vi "7FFT矩形窗校正子程序.vi"(6 "averaging parameters":T1={"averaging mode"=enum."No averaging", "weighting mode"=enum."Exponential", "number of averages"=10}, 7 "time signal":waveform(dbl) caption="时间信号") -> (0 "FFT幅值":cluster{"f0":dbl, "df":dbl, "magnitude":dbl[]}(graph), 2 "FFT相位":cluster{"f0":dbl, "df":dbl, "phase":dbl[]}(graph), 3 "频率":dbl)   [LabVIEW 2017]
uses:
  <vilib>/Analysis/4window.llb/windowTd.ctl
  <vilib>/measure/maspectr.llb/FFT Spectrum (Mag-Phase) for 1 Chan.vi
  <vilib>/measure/NI_MAPro.lvlib
  <vilib>/Analysis/NI_AALPro.lvlib
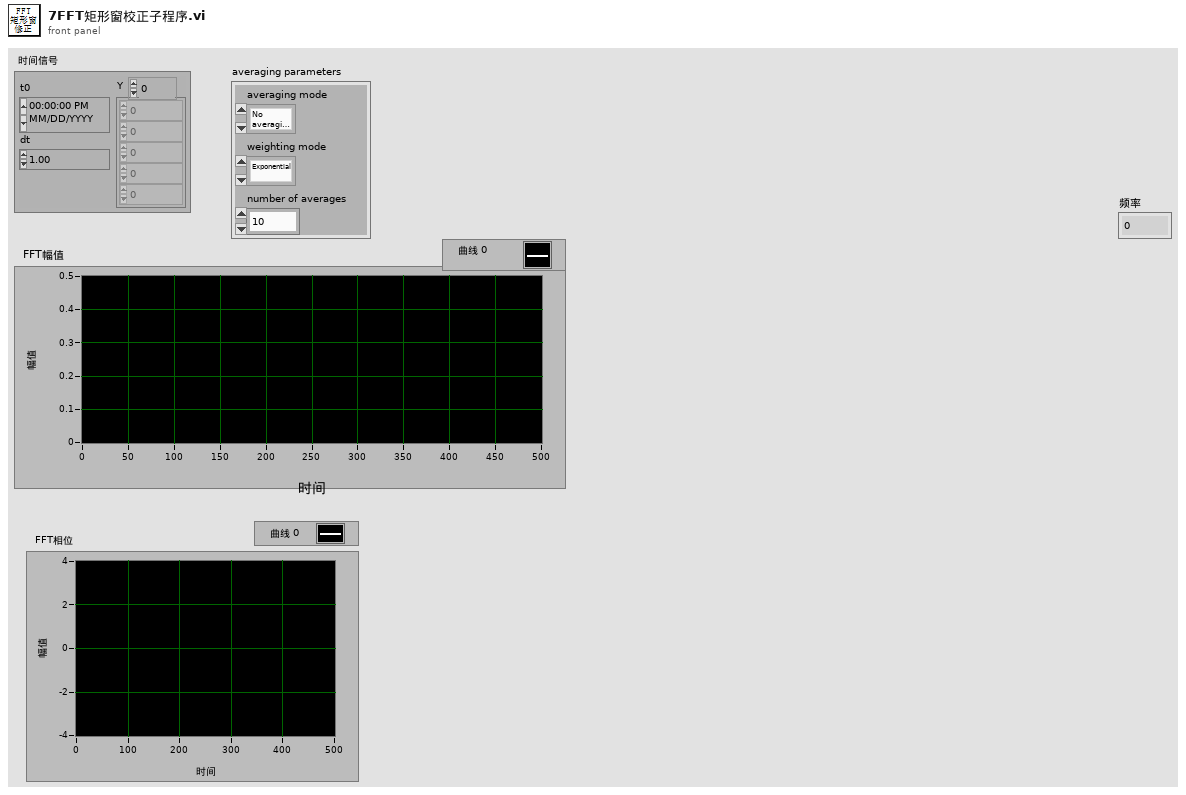
[diagram p1: front panel]
types:
  T1 = cluster{"averaging mode":enum16{"No averaging", "Vector averaging", "RMS averaging", "Peak hold"}, "weighting mode":enum16{"Linear", "Exponential"}, "number of averages":u32}
  T2 = typedef "NI_AALPro.lvlib/windowTd.ctl" = u32
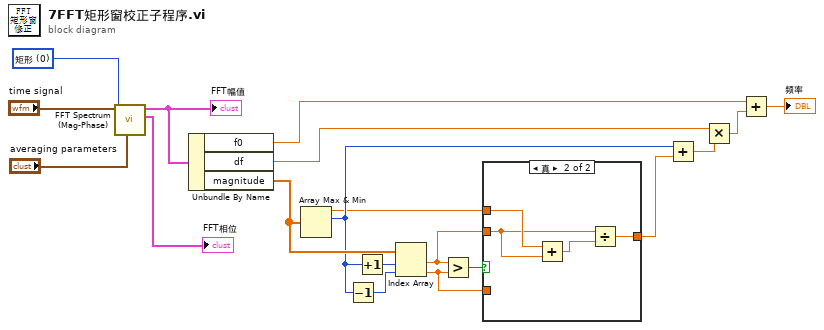
[diagram p0: block diagram]
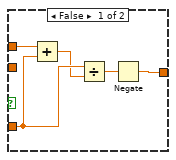
[diagram p2: hidden frame]
diagram:
  w17 = T2 0 items=["矩形"=0, "Hanning"=1, "Hamming"=2, "Blackman-Harris"=3, "Exact Blackman"=4, "Blackman"=5, "Flat Top"=6, "4阶Blackman-Harris "=7, "7阶Blackman-Harris"=8, "Low Sidelobe"=9, "Blackman Nuttall"=11, "三角"=30, "Bartlett-Hanning"=31, "Bohman"=32, "Parzen"=33, "Welch"=34, "Kaiser"=60, "Dolph-Chebyshev"=61, "高斯"=62] ("window")
  n1 = call-poly <vilib>:"FFT Spectrum (Mag-Phase).vi"("averaging parameters"="averaging parameters", "window"=w17, "time signal"="time signal") -> ("phase"=→"FFT相位":cluster{"f0":dbl, "df":dbl, "phase":dbl[]}, "magnitude"=w19:cluster{"f0":dbl, "df":dbl, "magnitude":dbl[]})  [unwired: 4 in, 3 out]
  "FFT幅值" <- w19
  n2 = Unbundle By Name(w19) -> ("f0"=w14:dbl, "df"=w8:dbl, "magnitude"=w13:dbl[])
  n3 = Array Max & Min(array=w13) -> (max value=w2:dbl, max index (indices)=w5:i32)  [unwired: 2 out]
  n4 = Decrement(x=w5) -> (x-1=w7:i32)
  n5 = Increment(x=w5) -> (x+1=w12:i32)
  n6 = Index Array(array=w13, index #1=w12, index #2=w7) -> (element #1=w4:dbl, element #2=w3:dbl)
  n7 = Greater?(x=w4, y=w3) -> (0:w6:bool)
  n8 = case shown="真" w6 {
    tunnel: w4 -> [_ w26]
    tunnel: w3 -> [w23 _]
    tunnel: w2 -> [w24 w28]
    tunnel: [w21 w25] -> w1
    frame False {
      n9 = Add(x=w24, y=w23) -> (x+y=w20:dbl)
      n10 = Divide(x=w23, y=w20) -> (x/y=w22:dbl)
      n11 = Negate(x=w22) -> (-x=w21:dbl)
    }
    frame True {
      n12 = Add(x=w28, y=w26) -> (x+y=w27:dbl)
      n13 = Divide(x=w26, y=w27) -> (x/y=w25:dbl)
    }
  }
  n14 = Add(x=w5, y=w1) -> (x+y=w11:dbl)
  n15 = Multiply(x=w8, y=w11) -> (x*y=w9:dbl)
  n16 = Add(x=w14, y=w9) -> (x+y=→"频率":dbl)
